vi "总磷氨氮测量数据储存.vi"   [LabVIEW 2016, in "氨氮总磷.lvlib"]
types:
  T1 = cluster{"时间标识":timestamp, "监测值":sgl, "单位":u16, "数据标识":string, "因子编码":u32, "标样参考值":sgl, "F0":sgl, "F1":sgl, "F2":sgl, "F3":sgl, "温度":sgl, "湿度":sgl, "量程标识":string}
  T2 = enum16{"维护数据", "水样测试", "标样核查", "零点核查", "跨度核查", "空白测试", "平行样测试", "加标回收", "空白校准", "标样校准", "初始化（清洗）"}
  T3 = cluster{"系统时间":timestamp, "工作状态":enum16{"空闲", "水样测试", "标样核查", "零点核查", "跨度核查", "空白测试", "平行样测试", "加标回收", "空白校准", "标样校准", "初始化（清洗）"}, "测量模式":enum16{"待机", "连续模式", "周期模式", "定点模式", "受控模式", "手动模式"}, "告警代码":enum16{"无告警", "缺试剂告警", "缺水样告警", "缺蒸馏水告警", "缺标液告警", "仪表漏液告警", "标定异常告警", "超量程告警", "加热异常", "低试剂预警", "超上限告警", "超下限告警", "仪表内部其他异常", "滴定异常告警", "电极异常告警", "量程切换告警", "参数设置告警", "PH电极电位异常", "电导率电极异常", "浊度光度异常", "溶解氧电极异常", "溶解氧光强异常", "温度异常告警", "PH异常告警", "溶解氧异常告警", "电导率异常告警", "浊度异常告警", "叶绿素异常告警", "藻密度异常告警", "蓝绿藻异常告警", "ORP异常告警", "氨氮异常告警", "清洁刷异常告警", "SD卡异常告警", "蓝牙异常告警", "Wifi异常告警", "流程异常告警"}, "故障代码":enum16{"无故障", "电机故障", "温度故障", "通讯故障", "滴定故障"}, "日志代码":u16, "软件版本":u16, "F0":sgl, "F1":sgl, "F2":sgl, "F3":sgl, "T":sgl, "H":sgl, "id":u16, "flowid":u16, "量程":u16, "总磷控温温度1":sgl, "营养盐控温温度2":sgl, "ADC":sgl}
  T4 = enum16{"空闲", "水样测试", "标样核查", "零点核查", "跨度核查", "空白测试", "平行样测试", "加标回收", "空白校准", "标样校准", "初始化（清洗）"}
  T5 = cluster{"因子编码":u32, "单位":u16, "标样参考值":sgl, "水样数据时间":timestamp, "水样实测值":sgl, "水样数据标识":string, "标样数据时间":timestamp, "标样实测值":sgl, "标样数据标识":string, "空白数据时间":timestamp, "空白实测值":sgl, "空白数据标识":string, "零点核查数据时间":timestamp, "零点核查实测值":sgl, "零点核查数据标识":string, "跨度核查数据时间":timestamp, "跨度核查实测值":sgl, "跨度核查数据标识":string, "加标回收数据时间":timestamp, "加标回收实测值":sgl, "加标回收数据标识":string, "平行样数据时间":timestamp, "平行样实测值":sgl, "平行样数据标识":string}
  T6 = cluster{"总磷跨度值":dbl, "总磷零点标准液浓度":dbl, "总磷跨度标准液浓度":dbl, "总磷标准液标准浓度":dbl, "氨氮跨度值":dbl, "氨氮零点标准液浓度":dbl, "氨氮跨度标准液浓度":dbl, "氨氮标准液标准浓度":dbl}
  T7 = cluster{"运行模式":enum16{"维护模式", "常规模式", "应急模式", "质控模式"}}
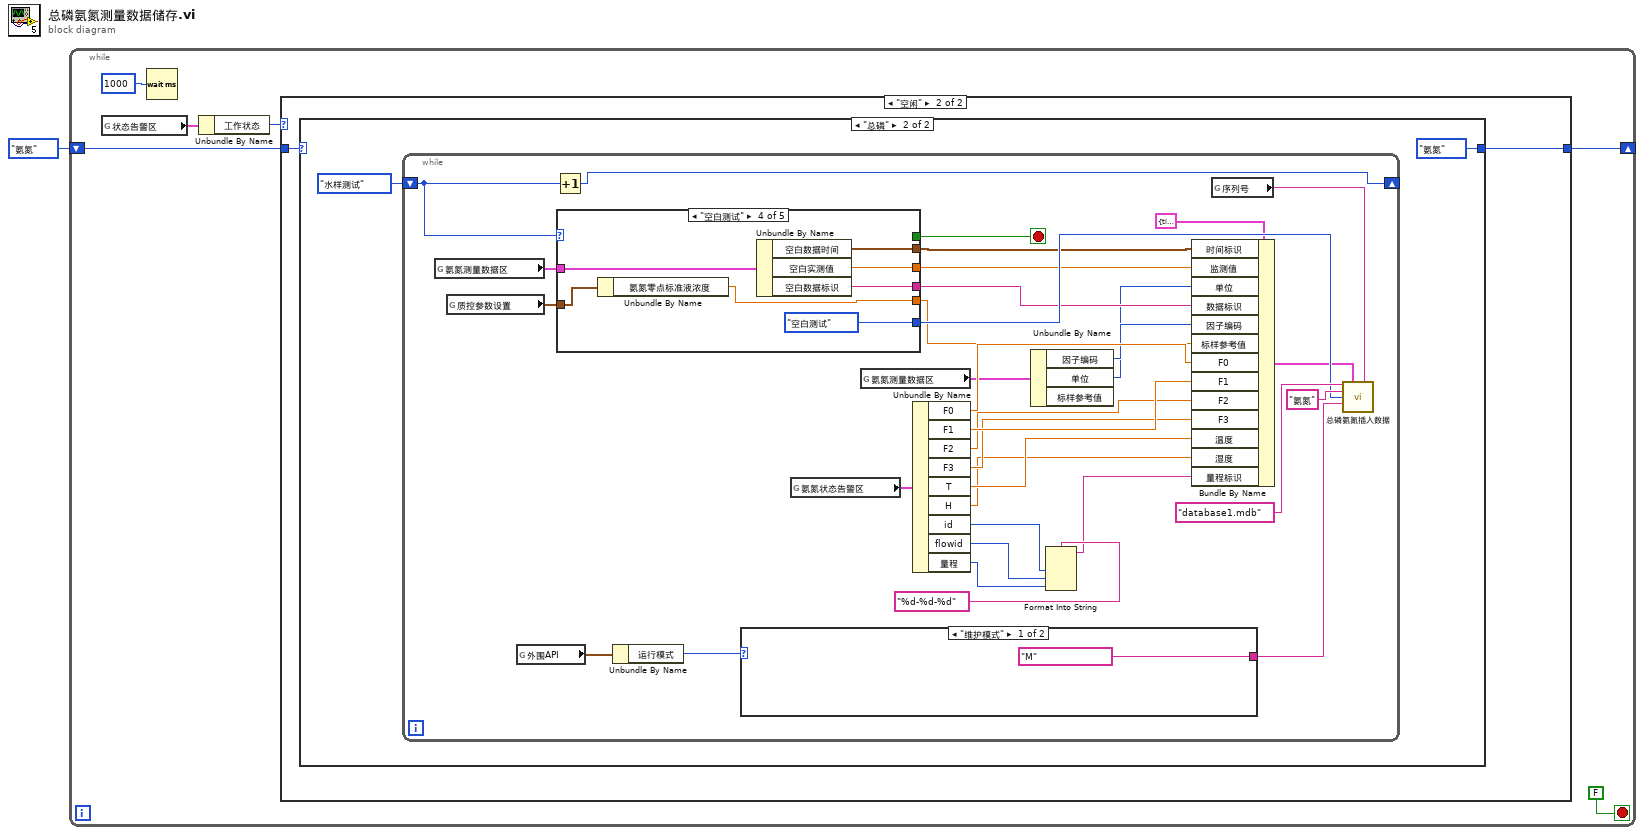
[diagram p0: block diagram]
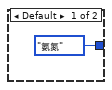
[diagram p2: hidden frame]
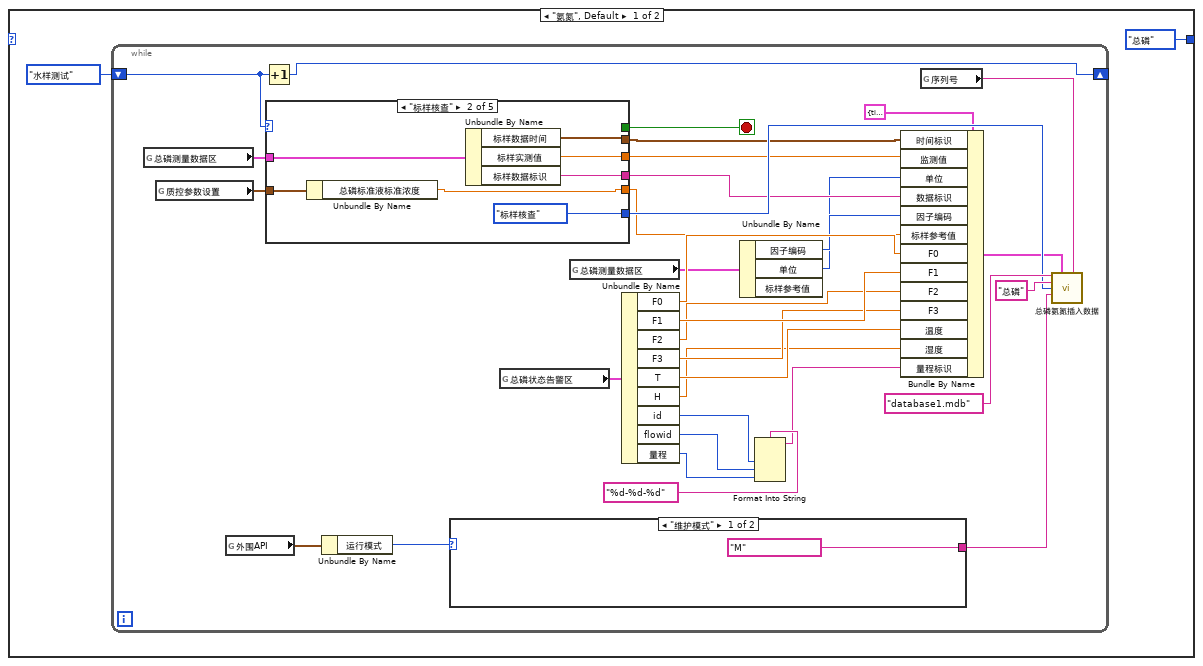
[diagram p3: hidden frame]
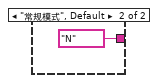
[diagram p4: hidden frame]
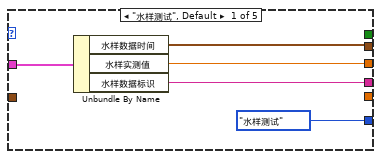
[diagram p5: hidden frame]
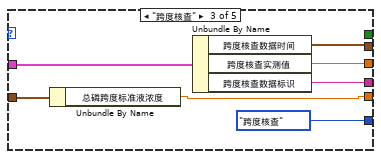
[diagram p6: hidden frame]
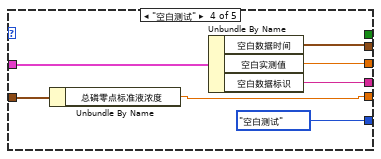
[diagram p7: hidden frame]
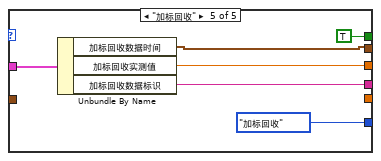
[diagram p8: hidden frame]
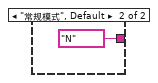
[diagram p9: hidden frame]
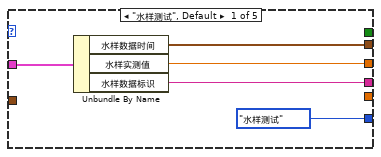
[diagram p10: hidden frame]
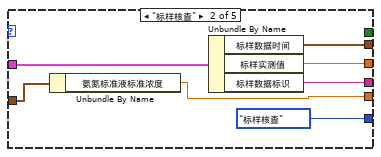
[diagram p11: hidden frame]
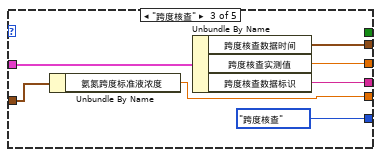
[diagram p12: hidden frame]
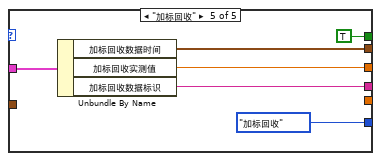
[diagram p13: hidden frame]
diagram:
  n1 = while {
    shift-right: [w2] -> _
    shift-left: enum16{"氨氮", "总磷"}."氨氮" ("测量模式") -> [w3]
    stop <- FALSE stop-if-true
    n2 = global read "VAR总磷氨氮全局变量.vi" "状态告警区"() -> (w5:T3)
    n3 = Wait (ms)(milliseconds to wait=u32 1000 ("等待时间（毫秒）")) -> ()  [unwired: 1 out]
    n4 = Unbundle By Name(w5) -> ("工作状态"=w4:T4)
    n5 = case shown="\"空闲\"" w4 {
      tunnel: w3 -> [_ w10]
      tunnel: [enum16{"氨氮", "总磷"}."氨氮" ("测量模式") w9] -> w2
      frame Default {
      }
      frame "空闲" {
        n6 = case shown="\"总磷\"" w10 {
          tunnel: [enum16{"氨氮", "总磷"}."总磷" ("测量模式") enum16{"氨氮", "总磷"}."氨氮" ("测量模式")] -> w9
          frame "氨氮", Default {
            n7 = while {
              shift-right: [w43] -> _
              shift-left: enum16{"水样测试", "标样核查", "跨度核查", "空白测试", "加标回收"}."水样测试" ("测量模式") -> [w44]
              stop <- w45 stop-if-true
              n8 = global read "VAR总磷氨氮全局变量.vi" "总磷测量数据区"() -> (w42:T5)
              n9 = global read "总磷氨氮断电保存全局变量.vi" "质控参数设置"() -> (w17:T6)
              n10 = global read "VAR总磷氨氮全局变量.vi" "外围API"() -> (w15:T7)
              n11 = Increment(x=w44) -> (x+1=w43:enum16{"水样测试", "标样核查", "跨度核查", "空白测试", "加标回收"})
              n12 = case shown="\"标样核查\"" w44 {
                tunnel: w42 -> [w52 w59 w66 w73 w79]
                tunnel: [w51 w58 w65 w72 w78] -> w35
                tunnel: [w50 w57 w64 w71 w77] -> w34
                tunnel: [w49 w56 w63 w70 w76] -> w33
                tunnel: [T2."水样测试" ("测量模式") T2."标样核查" ("测量模式") T2."跨度核查" ("测量模式") T2."空白测试" ("测量模式") T2."加标回收" ("测量模式")] -> w39
                tunnel: [_ _ _ _ TRUE] -> w45
                tunnel: w17 -> [_ w54 w61 w68 _]
                tunnel: [_ w53 w60 w67 _] -> w16
                frame "水样测试", Default {
                  n13 = Unbundle By Name(w52) -> ("水样数据时间"=w51:timestamp, "水样实测值"=w50:sgl, "水样数据标识"=w49:string)
                }
                frame "标样核查" {
                  n14 = Unbundle By Name(w54) -> ("总磷标准液标准浓度"=w53:dbl)
                  n15 = Unbundle By Name(w59) -> ("标样数据时间"=w58:timestamp, "标样实测值"=w57:sgl, "标样数据标识"=w56:string)
                }
                frame "跨度核查" {
                  n16 = Unbundle By Name(w61) -> ("总磷跨度标准液浓度"=w60:dbl)
                  n17 = Unbundle By Name(w66) -> ("跨度核查数据时间"=w65:timestamp, "跨度核查实测值"=w64:sgl, "跨度核查数据标识"=w63:string)
                }
                frame "空白测试" {
                  n18 = Unbundle By Name(w68) -> ("总磷零点标准液浓度"=w67:dbl)
                  n19 = Unbundle By Name(w73) -> ("空白数据时间"=w72:timestamp, "空白实测值"=w71:sgl, "空白数据标识"=w70:string)
                }
                frame "加标回收" {
                  n20 = Unbundle By Name(w79) -> ("加标回收数据时间"=w78:timestamp, "加标回收实测值"=w77:sgl, "加标回收数据标识"=w76:string)
                }
              }
              n21 = Unbundle By Name(w15) -> ("运行模式"=w14:enum16{"维护模式", "常规模式", "应急模式", "质控模式"})
              n22 = case shown="\"维护模式\"" w14 {
                tunnel: ["M" ("数据标记表") "N" ("数据标记表")] -> w13
                frame "维护模式" {
                }
                frame "常规模式", Default {
                }
              }
              n23 = global read "VAR总磷氨氮全局变量.vi" "总磷状态告警区"() -> (w32:T3)
              n24 = global read "VAR总磷氨氮全局变量.vi" "总磷测量数据区"() -> (w20:T5)
              n25 = Unbundle By Name(w32) -> ("F0"=w27:sgl, "F1"=w26:sgl, "F2"=w25:sgl, "F3"=w24:sgl, "T"=w23:sgl, "H"=w22:sgl, "id"=w30:u16, "flowid"=w29:u16, "量程"=w28:u16)
              n26 = Unbundle By Name(w20) -> ("因子编码"=w19:u32, "单位"=w18:u16)  [unwired: 1 out]
              n27 = Format Into String(format string="%d-%d-%d" ("格式字符串"), w30, w29, w28) -> (resulting string=w21:string)  [unwired: 2 in, 1 out]
              n28 = Bundle By Name(cluster=T1 {"时间标识"=timestamp(0 s since 1904-01-01), "监测值"=0.0, "单位"=0, "数据标识"="", "因子编码"=0, "标样参考值"=0.0, "F0"=0.0, "F1"=0.0, "F2"=0.0, "F3"=0.0, "温度"=0.0, "湿度"=0.0, "量程标识"=""} ("data"), "时间标识"=w35, "监测值"=w34, "单位"=w18, "数据标识"=w33, "因子编码"=w19, "标样参考值"=w16, "F0"=w27, "F1"=w26, "F2"=w25, "F3"=w24, "温度"=w23, "湿度"=w22, "量程标识"=w21) -> (w36:T1)
              n29 = global read "VAR总磷氨氮全局变量.vi" "序列号"() -> (w38:string)
              n30 = call "总磷氨氮插入数据.vi"("database"="database1.mdb", "data"=w36, "SN"=w38, "table"="总磷", "测量模式"=w39, "数据标记表"=w13) -> ()  [unwired: 9 in, 1 out]
            }
          }
          frame "总磷" {
            n31 = while {
              shift-right: [w112] -> _
              shift-left: enum16{"水样测试", "标样核查", "跨度核查", "空白测试", "加标回收"}."水样测试" ("测量模式") -> [w113]
              stop <- w114 stop-if-true
              n32 = global read "VAR总磷氨氮全局变量.vi" "氨氮测量数据区"() -> (w111:T5)
              n33 = global read "总磷氨氮断电保存全局变量.vi" "质控参数设置"() -> (w86:T6)
              n34 = global read "VAR总磷氨氮全局变量.vi" "外围API"() -> (w84:T7)
              n35 = Increment(x=w113) -> (x+1=w112:enum16{"水样测试", "标样核查", "跨度核查", "空白测试", "加标回收"})
              n36 = case shown="\"空白测试\"" w113 {
                tunnel: w111 -> [w117 w124 w131 w138 w143]
                tunnel: [w121 w128 w135 w142 w148] -> w92
                tunnel: [w120 w127 w134 w141 w147] -> w91
                tunnel: [w119 w126 w133 w140 w146] -> w90
                tunnel: [T2."水样测试" ("测量模式") T2."标样核查" ("测量模式") T2."跨度核查" ("测量模式") T2."空白测试" ("测量模式") T2."加标回收" ("测量模式")] -> w107
                tunnel: [_ _ _ _ TRUE] -> w114
                tunnel: w86 -> [_ w123 w130 w137 _]
                tunnel: [_ w122 w129 w136 _] -> w85
                frame "水样测试", Default {
                  n37 = Unbundle By Name(w117) -> ("水样数据时间"=w121:timestamp, "水样实测值"=w120:sgl, "水样数据标识"=w119:string)
                }
                frame "标样核查" {
                  n38 = Unbundle By Name(w123) -> ("氨氮标准液标准浓度"=w122:dbl)
                  n39 = Unbundle By Name(w124) -> ("标样数据时间"=w128:timestamp, "标样实测值"=w127:sgl, "标样数据标识"=w126:string)
                }
                frame "跨度核查" {
                  n40 = Unbundle By Name(w130) -> ("氨氮跨度标准液浓度"=w129:dbl)
                  n41 = Unbundle By Name(w131) -> ("跨度核查数据时间"=w135:timestamp, "跨度核查实测值"=w134:sgl, "跨度核查数据标识"=w133:string)
                }
                frame "空白测试" {
                  n42 = Unbundle By Name(w137) -> ("氨氮零点标准液浓度"=w136:dbl)
                  n43 = Unbundle By Name(w138) -> ("空白数据时间"=w142:timestamp, "空白实测值"=w141:sgl, "空白数据标识"=w140:string)
                }
                frame "加标回收" {
                  n44 = Unbundle By Name(w143) -> ("加标回收数据时间"=w148:timestamp, "加标回收实测值"=w147:sgl, "加标回收数据标识"=w146:string)
                }
              }
              n45 = Unbundle By Name(w84) -> ("运行模式"=w83:enum16{"维护模式", "常规模式", "应急模式", "质控模式"})
              n46 = case shown="\"维护模式\"" w83 {
                tunnel: ["M" ("数据标记表") "N" ("数据标记表")] -> w82
                frame "维护模式" {
                }
                frame "常规模式", Default {
                }
              }
              n47 = global read "VAR总磷氨氮全局变量.vi" "氨氮状态告警区"() -> (w106:T3)
              n48 = global read "VAR总磷氨氮全局变量.vi" "氨氮测量数据区"() -> (w89:T5)
              n49 = Unbundle By Name(w106) -> ("F0"=w105:sgl, "F1"=w104:sgl, "F2"=w103:sgl, "F3"=w102:sgl, "T"=w101:sgl, "H"=w100:sgl, "id"=w98:u16, "flowid"=w97:u16, "量程"=w96:u16)
              n50 = Unbundle By Name(w89) -> ("因子编码"=w88:u32, "单位"=w87:u16)  [unwired: 1 out]
              n51 = Format Into String(format string="%d-%d-%d" ("格式字符串"), w98, w97, w96) -> (resulting string=w94:string)  [unwired: 2 in, 1 out]
              n52 = Bundle By Name(cluster=T1 {"时间标识"=timestamp(0 s since 1904-01-01), "监测值"=0.0, "单位"=0, "数据标识"="", "因子编码"=0, "标样参考值"=0.0, "F0"=0.0, "F1"=0.0, "F2"=0.0, "F3"=0.0, "温度"=0.0, "湿度"=0.0, "量程标识"=""} ("data"), "时间标识"=w92, "监测值"=w91, "单位"=w87, "数据标识"=w90, "因子编码"=w88, "标样参考值"=w85, "F0"=w105, "F1"=w104, "F2"=w103, "F3"=w102, "温度"=w101, "湿度"=w100, "量程标识"=w94) -> (w93:T1)
              n53 = global read "VAR总磷氨氮全局变量.vi" "序列号"() -> (w110:string)
              n54 = call "总磷氨氮插入数据.vi"("database"="database1.mdb", "data"=w93, "SN"=w110, "table"="氨氮", "测量模式"=w107, "数据标记表"=w82) -> ()  [unwired: 9 in, 1 out]
            }
          }
        }
      }
    }
  }
